vi "Colour Recognition.vi"() -> ()   [LabVIEW 2013]
uses:
  <vilib>/userdefined/High Color/IMAQdx.ctl
  <vilib>/vision/driver/NI_Vision_Acquisition_Software.lvlib
  <vilib>/vision/NI_Vision_Development_Module.lvlib
panel:
  in  "Reset Default Settings":bool
  in  "Threshold":cluster{"Lower value":sgl, "Upper value":sgl}={"Lower value"=125.0, "Upper value"=160.0} {"Lower value" scale=0.0..255.0; "Upper value" scale=0.0..255.0}
  in  "Color Recognition":enum16{"Blue", "Red"}(ring)
  out "Image Preview":T1(plugin-control)
  in  "Erosion Value":dbl=5.0
  out "Object Area":dbl
  in  "Area Limit":dbl=2000.0 format="%#_13g"
  out "Colour Matching":T1(plugin-control)
  in  "STOP":bool
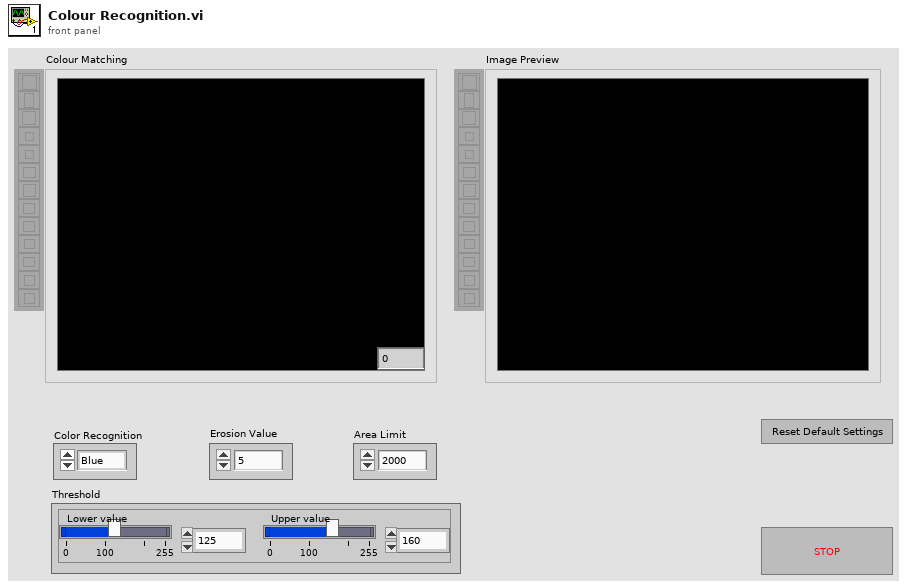
[diagram p1: front panel]
types:
  T1 = typedef "IMAQ Image.ctl" = refnum<image>
  T2 = typedef "IMAQdx.ctl" = refnum<k21>
  T3 = typedef "Particle Parameters" = i32
  T4 = cluster{"Numeric":dbl, "Numeric":dbl, "Numeric":dbl, "Numeric":dbl}
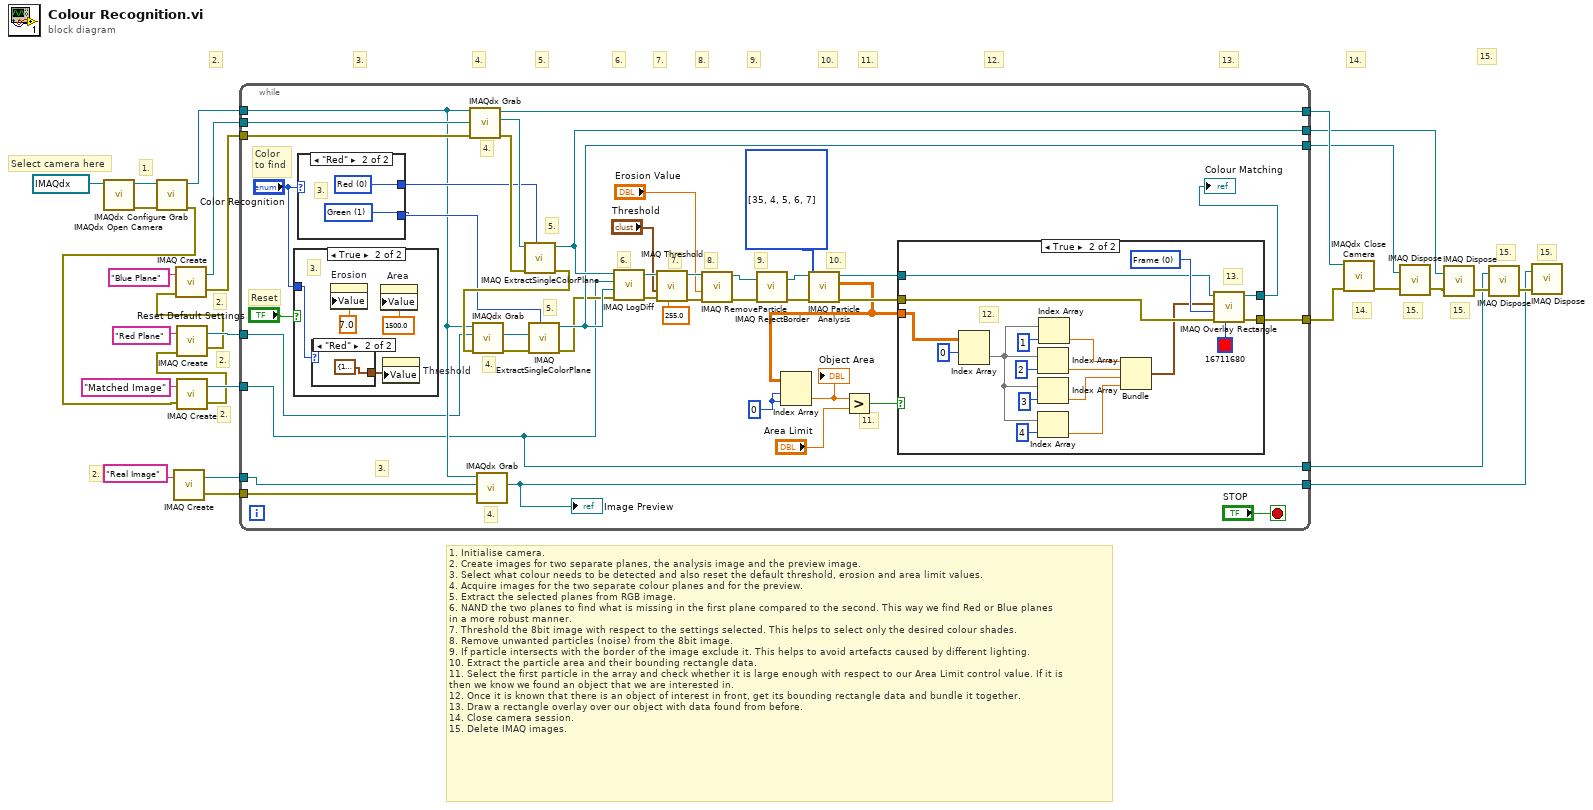
[diagram p0: block diagram]
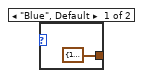
[diagram p3: hidden frame]
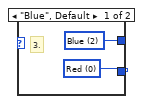
[diagram p4: hidden frame]
diagram:
  # "Select camera here"
  # "1. Initialise camera.\n2. Create images for two separate planes, the analysis image and the preview image.\n3. Select what colour needs to be detected and also reset the default threshold, erosion and area limit values.\n4. Acquire images for the two separate colour planes and for the preview.\n5. Extract the selected planes from RGB image.\n6. NAND the two planes to find what is missing in the first plane compared to the second. This way we find Red or Blue planes\nin a more robust manner.\n7. Threshold the 8bit image with respect to the settings selected. This helps to select only the desired colour shades.\n8. Remove unwanted particles (noise) from the 8bit image.\n9. If particle intersects with the border of the image exclude it. This helps to avoid artefacts caused by different lighting.\n10. Extract the particle area and their bounding rectangle data.\n11. Select the first particle in the array and check whether it is large enough with respect to our Area Limit control value. If it is\nthen we know we found an object that we are interested in.\n12. Once it is known that there is an object of interest in front, get its bounding rectangle data and bundle it together.\n13. Draw a rectangle overlay over our object with data found from before.\n14. Close camera session.\n15. Delete IMAQ images."
  # "15."
  # "15."
  # "15."
  # "15."
  # "15."
  # "14."
  # "14."
  # "13."
  # "12."
  # "11."
  # "10."
  # "2."
  # "2."
  # "2."
  # "2."
  # "9."
  # "8."
  # "7."
  # "6."
  # "5."
  # "4."
  # "3."
  # "2."
  # "1."
  n1 = call <vilib>:"IMAQdx Open Camera.vi"("Session In"=T2 "cam1") -> ("error out"=w22:errorcluster, "Session Out"=w23:T2)  [unwired: 9 in]
  n2 = call <vilib>:"IMAQdx Configure Grab.vi"("error in"=w22, "Session In"=w23) -> ("error out"=w9:errorcluster, "Session Out"=w21:T2)  [unwired: 8 in]
  n3 = call "IMAQ Create"("Image Name"="Real Image") -> ("New Image"=w4:T1, "error out"=w3:errorcluster)  [unwired: 3 in, 1 out]
  n4 = call "IMAQ Create"("Image Name"="Matched Image", "error in (no error)"=w9) -> ("New Image"=w14:T1, "error out"=w8:errorcluster)  [unwired: 2 in, 1 out]
  n5 = call "IMAQ Create"("Image Name"="Red Plane", "error in (no error)"=w8) -> ("New Image"=w17:T1, "error out"=w7:errorcluster)  [unwired: 2 in, 1 out]
  n6 = call "IMAQ Create"("Image Name"="Blue Plane", "error in (no error)"=w7) -> ("New Image"=w26:T1, "error out"=w25:errorcluster)  [unwired: 2 in, 1 out]
  n7 = while {
    tunnel: w26 -> [w70]
    tunnel: w25 -> [w69]
    tunnel: w21 -> [w31]
    tunnel: [w65] -> w19
    tunnel: w17 -> [w30]
    tunnel: [w60] -> w10
    tunnel: [w59] -> w11
    tunnel: w14 -> [w29]
    tunnel: [w29] -> w6
    tunnel: [w46] -> w12
    tunnel: w4 -> [w39]
    tunnel: w3 -> [w37]
    tunnel: [w28] -> w1
    stop <- "STOP" stop-if-true
    w57 = 0 ("index (row)")
    w61 = T3[] [35, 4, 5, 6, 7] items=["Center of Mass X", "Center of Mass Y", "First Pixel X", "First Pixel Y", "Bounding Rect Left", "Bounding Rect Top", "Bounding Rect Right", "Bounding Rect Bottom", "Max Feret Diameter Start X", "Max Feret Diameter Start Y", "Max Feret Diameter End X", "Max Feret Diameter End Y", "Max Horiz. Segment Length Left", "Max Horiz. Segment Length Right", "Max Horiz. Segment Length Row", "-", "Bounding Rect Width", "Bounding Rect Height", "Bounding Rect Diagonal", "Perimeter", "Convex Hull Perimeter", "Holes' Perimeter", "Max Feret Diameter", "Equivalent Ellipse Major Axis", "Equivalent Ellipse Minor Axis", "Equivalent Ellipse Minor Axis (Feret)", "Equivalent Rect Long Side", "Equivalent Rect Short Side", "Equivalent Rect Diagonal", "Equivalent Rect Short Side (Feret)", "Average Horiz. Segment Length", "Average Vert. Segment Length", "Hydraulic Radius", "Waddel Disk Diameter", "-", "Area", "Holes' Area", "Particle & Holes' Area", "Convex Hull Area", "Image Area", "-", "Number of Holes", "Number of Horiz. Segments", "Number of Vert. Segments", "-", "Orientation", "Max Feret Diameter Orientation", "-", "% Area/Image Area", "% Area/(Particle & Holes' Area)", "Ratio of Equivalent Ellipse Axes", "Ratio of Equivalent Rect Sides", "-", "Elongation Factor", "Compactness Factor", "Heywood Circularity Factor", "Type Factor", "-", "Sum X", "Sum Y", "Sum XX", "Sum XY", "Sum YY", "Sum XXX", "Sum XXY", "Sum XYY", "Sum YYY", "-", "Moment of Inertia XX", "Moment of Inertia XY", "Moment of Inertia YY", "Moment of Inertia XXX", "Moment of Inertia XXY", "Moment of Inertia XYY", "Moment of Inertia YYY", "Norm. Moment of Inertia XX", "Norm. Moment of Inertia XY", "Norm. Moment of Inertia YY", "Norm. Moment of Inertia XXX", "Norm. Moment of Inertia XXY", "Norm. Moment of Inertia XYY", "Norm. Moment of Inertia YYY", "Hu Moment 1", "Hu Moment 2", "Hu Moment 3", "Hu Moment 4", "Hu Moment 5", "Hu Moment 6", "Hu Moment 7"] ("Pixel Measurements")
    # "3."
    # "11."
    # "10."
    # "4."
    # "4."
    # "4."
    # "5."
    # "5."
    # "6."
    # "7."
    # "8."
    # "9."
    # "Reset"
    # "Color\nto find"
    n8 = case shown="True" "Reset Default Settings" {
      tunnel: "Color Recognition" -> [_ w74]
      frame False {
        # "3."
      }
      frame True {
        # "3."
        n9 = case shown="\"Red\"" w74 {
          tunnel: [cluster{"Lower value":sgl, "Upper value":sgl} {"Lower value"=125.0, "Upper value"=160.0} ("Threshold Range") cluster{"Lower value":sgl, "Upper value":sgl} {"Lower value"=125.0, "Upper value"=137.0} ("Threshold Range")] -> w73
          frame "Blue", Default {
          }
          frame "Red" {
          }
        }
        n10 = property on="Erosion" class="DigNum (strict)"("Value"=7.0 ("Erosion Value")) -> ()  [unwired: 2 in, 2 out]
        n11 = property on="Area" class="DigNum (strict)"("Value"=1500.0 ("Area Limit")) -> ()  [unwired: 2 in, 2 out]
        n12 = property on="Threshold" class="Clust (strict)"("Value"=w73) -> ()  [unwired: 2 in, 2 out]
      }
    }
    n13 = case shown="\"Red\"" "Color Recognition" {
      tunnel: [w78 w80] -> w36
      tunnel: [w77 w79] -> w35
      frame "Blue", Default {
        w77 = 0 items=["Red", "Green", "Blue", "Hue", "Saturation", "Luminance", "Value", "Intensity"] ("Color Plane")
        w78 = 2 items=["Red", "Green", "Blue", "Hue", "Saturation", "Luminance", "Value", "Intensity"] ("Color Plane")
        # "3."
      }
      frame "Red" {
        w79 = 1 items=["Red", "Green", "Blue", "Hue", "Saturation", "Luminance", "Value", "Intensity"] ("Color Plane")
        w80 = 0 items=["Red", "Green", "Blue", "Hue", "Saturation", "Luminance", "Value", "Intensity"] ("Color Plane")
        # "3."
      }
    }
    n14 = call <vilib>:"IMAQdx Grab.vi"("error in"=w69, "Image In"=w70, "Session In"=w31) -> ("error out"=w45:errorcluster, "Image Out"=w40:T1, "Session Out"=w65:T2)  [unwired: 5 in, 1 out]
    n15 = call <vilib>:"IMAQdx Grab.vi"("error in"=w37, "Image In"=w39, "Session In"=w31) -> ("Image Out"=w28:T1)  [unwired: 5 in, 3 out]
    "Image Preview" <- w28
    n16 = call "IMAQ ExtractSingleColorPlane"("Color Plane"=w36, "error in (no error)"=w45, "Image Src"=w40) -> ("error out"=w44:errorcluster, "Image Dst Out"=w60:T1)  [unwired: 7 in]
    n17 = call <vilib>:"IMAQdx Grab.vi"("error in"=w44, "Image In"=w30, "Session In"=w31) -> ("error out"=w67:errorcluster, "Image Out"=w66:T1)  [unwired: 5 in, 2 out]
    n18 = call "IMAQ ExtractSingleColorPlane"("Color Plane"=w35, "error in (no error)"=w67, "Image Src"=w66) -> ("error out"=w38:errorcluster, "Image Dst Out"=w59:T1)  [unwired: 7 in]
    n19 = call "IMAQ LogDiff"("Image Src A"=w60, "Image Dst"=w29, "Image Src B"=w59, "error in (no error)"=w38) -> ("Image Dst Out"=w64:T1, "error out"=w63:errorcluster)  [unwired: 3 in]
    n20 = call "IMAQ Threshold"("Replace Value"=sgl 255.0, "error in (no error)"=w63, "Range"="Threshold", "Image Src"=w64) -> ("error out"=w52:errorcluster, "Image Dst Out"=w53:T1)  [unwired: 6 in]
    n21 = call "IMAQ RemoveParticle"("error in (no error)"=w52, "Number of Erosion"="Erosion Value", "Image Src"=w53) -> ("error out"=w51:errorcluster, "Image Dst Out"=w50:T1)  [unwired: 7 in]
    n22 = call "IMAQ RejectBorder"("error in (no error)"=w51, "Image Src"=w50) -> ("error out"=w48:errorcluster, "Image Dst Out"=w49:T1)  [unwired: 4 in]
    n23 = call "IMAQ Particle Analysis"("error in (no error)"=w48, "Pixel Measurements"=w61, "Image"=w49) -> ("error out"=w47:errorcluster, "Particle Measurements (Pixels)"=w43:dbl[][], "Image Out (duplicate)"=w58:T1)  [unwired: 3 in, 3 out]
    n24 = Index Array(array=w43, index (row)=w57, index (col)=w57) -> (element=w56:dbl)
    "Object Area" <- w56
    n25 = Greater?(x=w56, y="Area Limit") -> (0:w54:bool)
    n26 = case shown="True" w54 {
      tunnel: [w82 w99] -> w42
      tunnel: w58 -> [w82 w97]
      tunnel: w47 -> [w81 w93]
      tunnel: [w81 w96] -> w46
      tunnel: w43 -> [_ w95]
      frame False {
      }
      frame True {
        w98 = u32 0 items=["Frame", "Fill", "Highlight"] ("Drawing Mode (Frame)")
        # "13."
        # "12."
        n27 = Index Array(array=w95, index (row)=0) -> (element=w92:dbl[])  [unwired: 1 in]
        n28 = Index Array(array=w92, index=2) -> (element=w86:dbl)
        n29 = Index Array(array=w92, index=3) -> (element=w85:dbl)
        n30 = Index Array(array=w92, index=4) -> (element=w84:dbl)
        n31 = Index Array(array=w92, index=1) -> (element=w87:dbl)
        n32 = Bundle("Numeric"=w87, "Numeric"=w86, "Numeric"=w85, "Numeric"=w84) -> (w83:T4)  [unwired: 1 in]
        n33 = call "IMAQ Overlay Rectangle"("Color"=u32 16711680, "error in (no error)"=w93, "Drawing Mode (Frame)"=w98, "Rectangle"=w83, "Image"=w97) -> ("error out"=w96:errorcluster, "Image Out"=w99:T1)  [unwired: 5 in]
      }
    }
    "Colour Matching" <- w42
  }
  n34 = call <vilib>:"IMAQdx Close Camera.vi"("error in"=w12, "Session In"=w19) -> ("error out"=w20:errorcluster)  [unwired: 9 in]
  n35 = call "IMAQ Dispose"("Image"=w11, "error in (no error)"=w20) -> ("error out"=w16:errorcluster)  [unwired: 1 in, 3 out]
  n36 = call "IMAQ Dispose"("Image"=w10, "error in (no error)"=w16) -> ("error out"=w13:errorcluster)  [unwired: 1 in, 3 out]
  n37 = call "IMAQ Dispose"("Image"=w6, "error in (no error)"=w13) -> ("error out"=w2:errorcluster)  [unwired: 1 in, 3 out]
  n38 = call "IMAQ Dispose"("Image"=w1, "error in (no error)"=w2) -> ()  [unwired: 1 in, 4 out]
